vi "Job Completion Times.vi"(9 "Number Of Machines":i32=4, 10 "Number Of Jobs":i32=4, 11 "Gannt Chart In":T1[][](array[typedef])) -> (3 "Job Completion Times":u16[](array[numeric]))   [LabVIEW 2013, in "Scheduler.lvclass"]
uses:
  Scheduler.lvclass
  Controls/GanntChart_Element.ctl
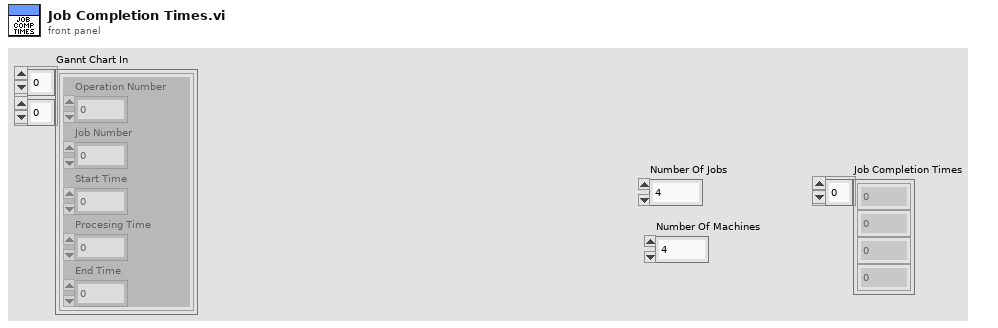
[diagram p1: front panel]
types:
  T1 = typedef "GanntChart_Element.ctl" = cluster{"Operation Number":i32, "Job Number":i32, "Start Time":i32, "Procesing Time":u16, "End Time":i32}
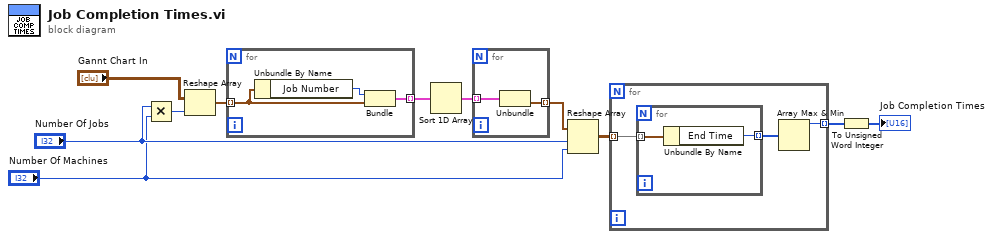
[diagram p0: block diagram]
diagram:
  n1 = Multiply(x="Number Of Jobs", y="Number Of Machines") -> (x*y=w6:i32)
  n2 = Reshape Array("Gannt Chart In", w6) -> (w11:T1[])
  n3 = for {
    tunnel: w11 -> [w13] mode=indexing
    tunnel: [w12] -> w10 mode=indexing
    n4 = Unbundle By Name(w13) -> ("Job Number"=w14:i32)
    n5 = Bundle("Job Number"=w14, w13) -> (w12:cluster{"Job Number":i32, T1})  [unwired: 1 in]
  }
  n6 = Sort 1D Array(array=w10) -> (sorted array=w9:cluster{"Job Number":i32, T1}[])
  n7 = for {
    tunnel: w9 -> [w16] mode=indexing
    tunnel: [w15] -> w8 mode=indexing
    n8 = Unbundle(w16) -> (w15:T1)  [unwired: 1 out]
  }
  n9 = Reshape Array(w8, "Number Of Jobs", "Number Of Machines") -> (w7:T1[][])
  n10 = for {
    tunnel: w7 -> [w19] mode=indexing
    tunnel: [w17] -> w3 mode=indexing
    n11 = for {
      tunnel: w19 -> [w21] mode=indexing
      tunnel: [w20] -> w18 mode=indexing
      n12 = Unbundle By Name(w21) -> ("End Time"=w20:i32)
    }
    n13 = Array Max & Min(array=w18) -> (max value=w17:i32)  [unwired: 3 out]
  }
  n14 = To Unsigned Word Integer(number=w3) -> (unsigned 16bit integer=→"Job Completion Times":u16[])
